vi "Add Stimulus Output Rows.vi"(8 "error in (no error)":errorcluster, 11 "Settings":T1 {"Processing Settings"."Test Parameters"."Allowed Tolerance (%) FS" format="%#_4g"; "Acq Settings"."Config Settings"."Simulated Sensor Injection" scale=0.0..100.0}) -> (0 "error out":errorcluster, 3 "Stimulus Outputs":T26)   [LabVIEW 2026, in "Settings.lvlib"]
uses:
  Settings.lvlib
  controls/UI/Stimulus Outputs Display.ctl
  controls/Controller/Stimulus Role.ctl
  controls/Controller/Stimulus Output Configuration.ctl
  controls/UI/Stimulus Output Display.ctl
  controls/UI/Measurement Role.ctl
  Acquisition/Instrument Specifications Cluster Configuration.ctl
  Acquisition/Acquisition.lvlib
  Acquisition/Instrument Specifications Configuration.ctl
  controls/UI/Config Settings.ctl
  controls/UI/Acq Settings.ctl
  controls/UI/Units Enum.ctl
  controls/UI/Signal Enum.ctl
  controls/Messaging Payloads/Sensor CoreData Cluster.ctl
  controls/Messaging Payloads/Sensor CoreData.ctl
  Processing/Test Parameters Cluster.ctl
  Processing/Test Parameters.ctl
  Processing/Processing_Engine.lvlib
  controls/UI/Direction.ctl
  controls/UI/Test Sequence Context.ctl
  Processing/Processing Settings.ctl
  controls/UI/Session Identfiers.ctl
  controls/UI/Test Sequence Enum.ctl
  controls/UI/Test Sequence State.ctl
  controls/UI/Test Sequence Settings.ctl
  controls/Controller/Controller Core Data.ctl
  controls/Controller/Stimulus Output.ctl
  controls/Controller/Stimulus Outputs.ctl
  controls/Controller/Stimulus Settings.ctl
  controls/UI/Settings Cluster.ctl
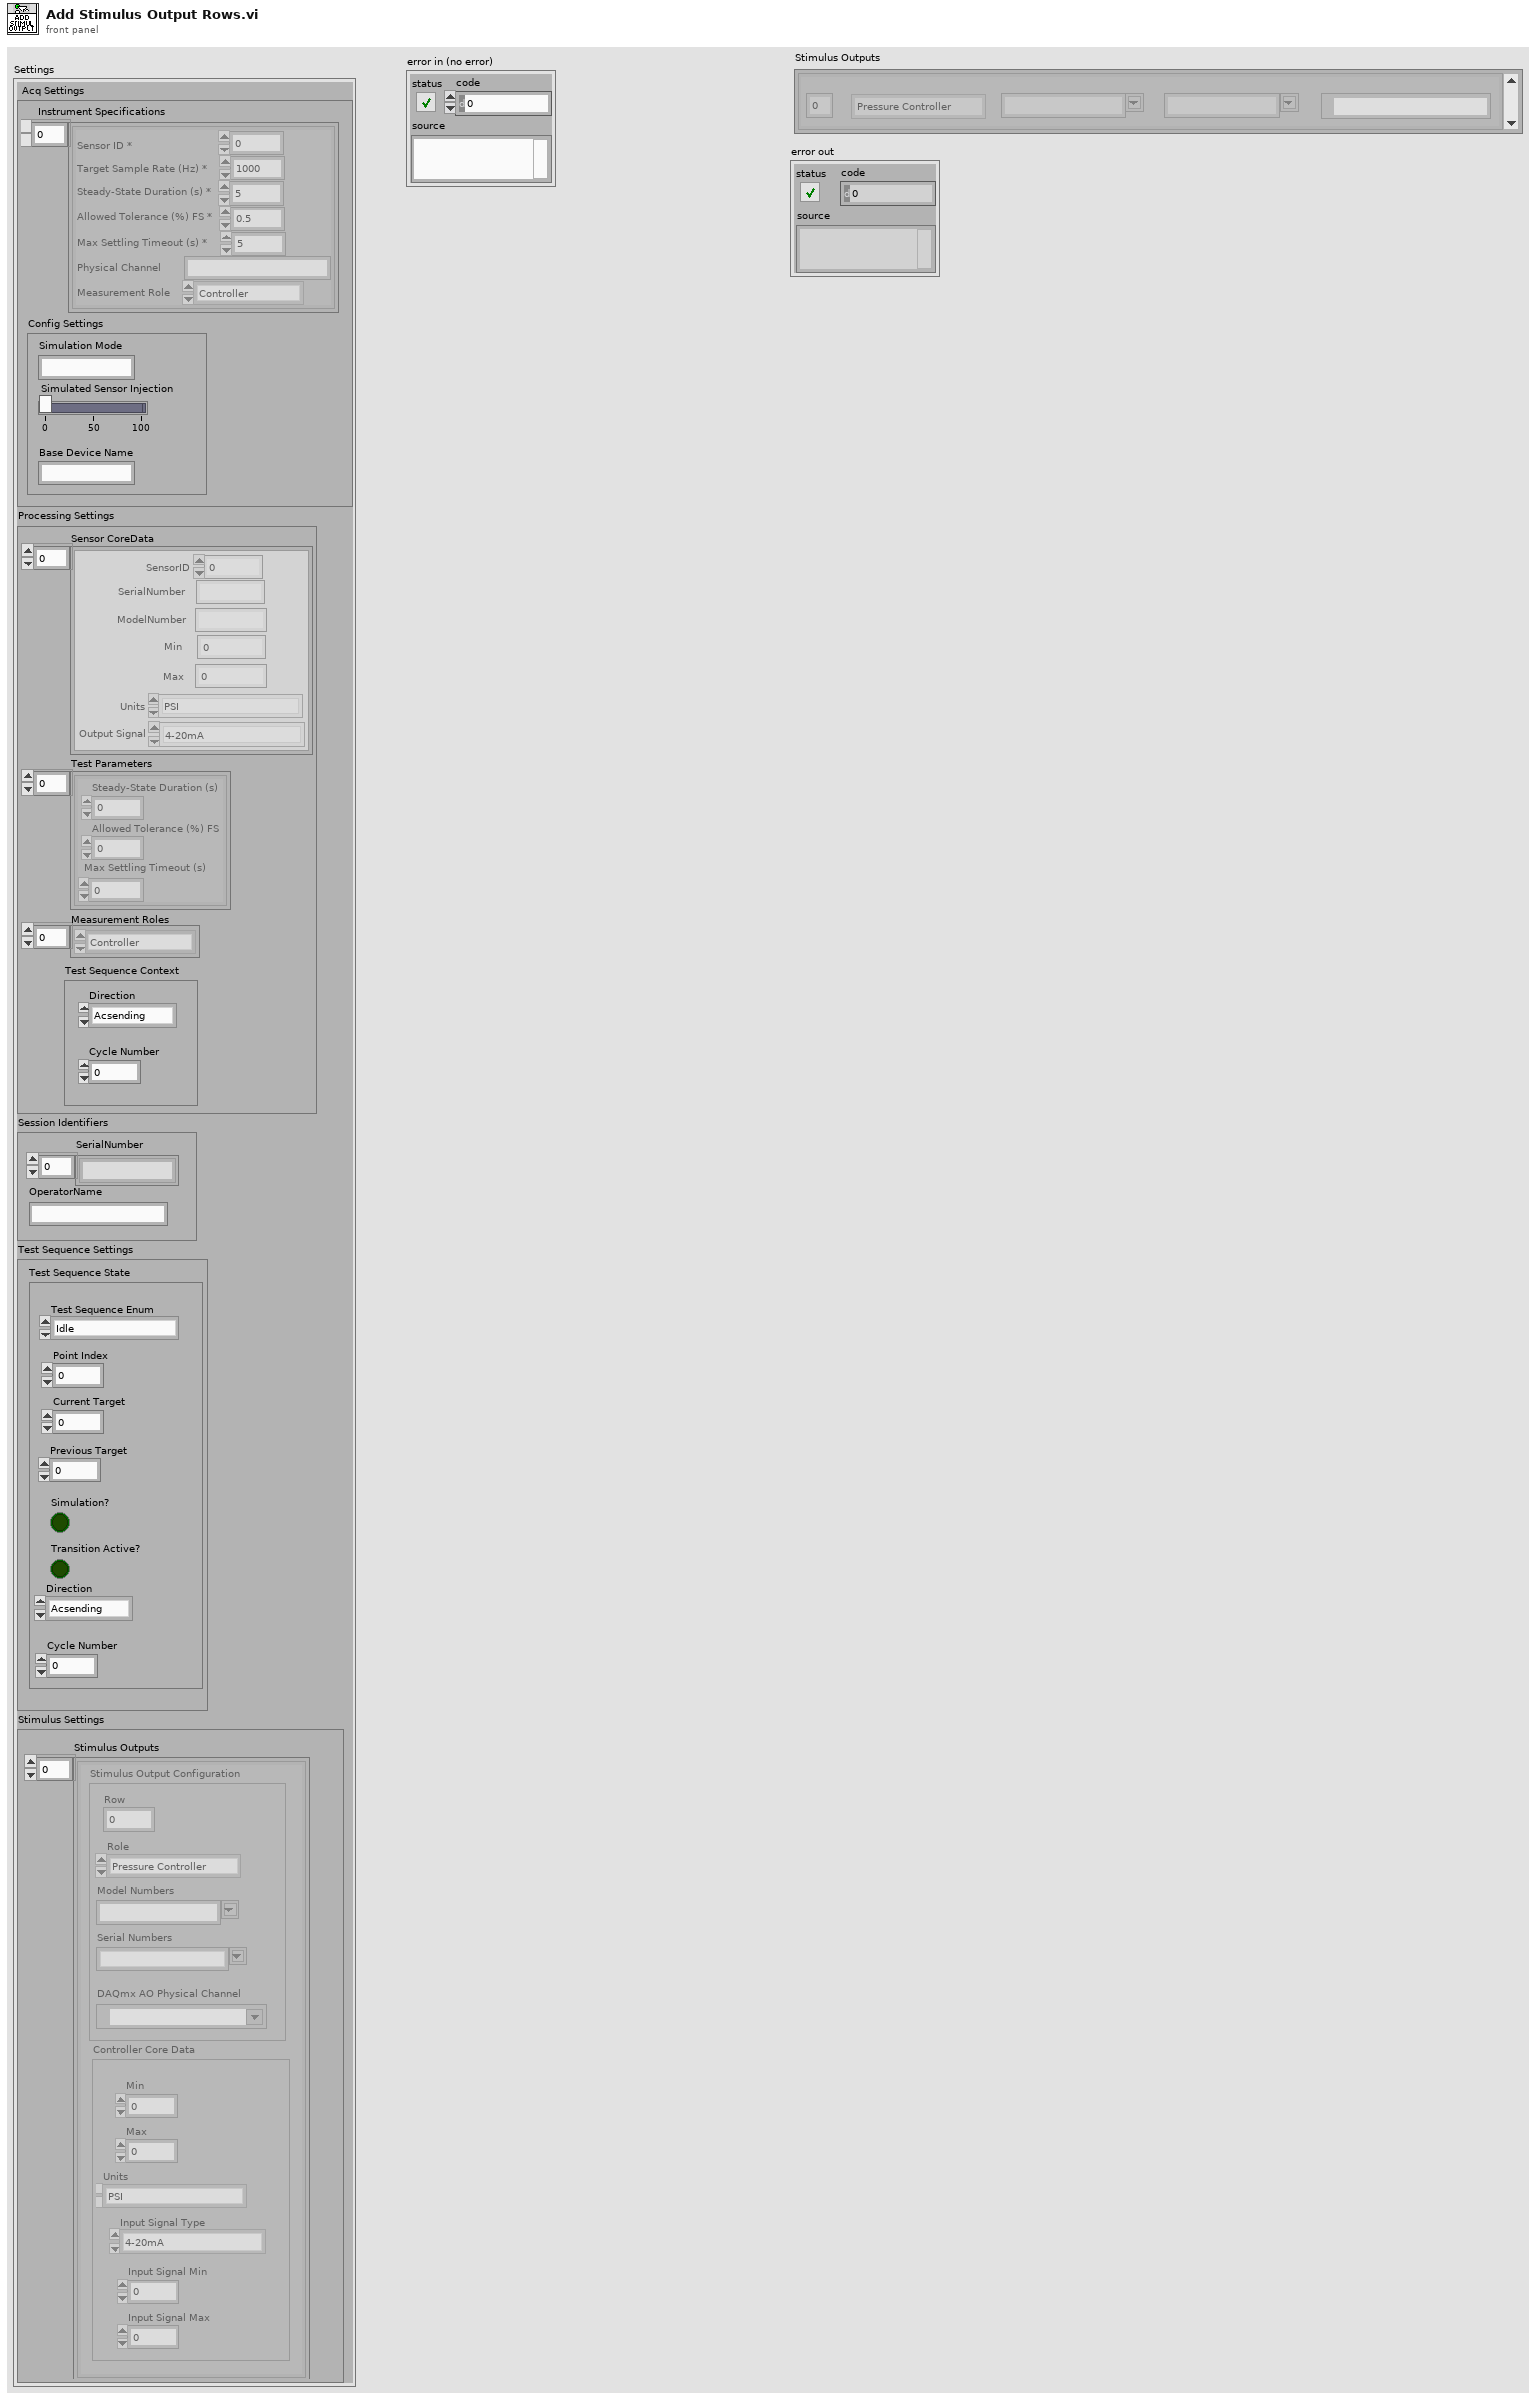
[diagram p1: front panel]
types:
  T1 = typedef "Settings Cluster.ctl" = cluster{"Acq Settings":T2, "Processing Settings":T7, "Session Identifiers":T16, "Test Sequence Settings":T17, "Stimulus Settings":T20}
  T2 = typedef "Acq Settings.ctl" = cluster{"Instrument Specifications":T3, "Config Settings":T6}
  T3 = typedef "Acquisition.lvlib/Instrument Specifications Configuration.ctl" = T4[]
  T4 = typedef "Acquisition.lvlib/Instrument Specifications Cluster Configuration.ctl" = cluster{"Sensor ID *":i32, "Target Sample Rate (Hz) *":dbl, "Steady-State Duration (s) *":i32, "Allowed Tolerance (%) FS *":dbl, "Max Settling Timeout (s) *":i32, "Physical Channel":string, "Measurement Role":T5}
  T5 = typedef "Settings.lvlib/Measurement Role.ctl" = enum16{"Controller", "Reference", "UUT", "Disable", "All"}
  T6 = typedef "Config Settings.ctl" = cluster{"Simulated Sensor Injection":dbl, "Base Device Name":string, "Simulation Mode":string}
  T7 = typedef "Processing_Engine.lvlib/Processing Settings.ctl" = cluster{"Sensor CoreData":T8, "Test Parameters":T12, "Measurement Roles":T5[], "Test Sequence Context":T14}
  T8 = typedef "Sensor CoreData.ctl" = T9[]
  T9 = typedef "Settings.lvlib/Sensor CoreData Cluster.ctl" = cluster{"SerialNumber":string, "ModelNumber":string, "Min":dbl, "Max":dbl, "Units":T10, "Output Signal":T11, "SensorID":i32}
  T10 = typedef "Units Enum.ctl" = enum16{"PSI", "Deg C", "kPa", "GPM"}
  T11 = typedef "Signal Enum.ctl" = enum16{"4-20mA", "0-10V", "Thermocouple Type K"}
  T12 = typedef "Processing_Engine.lvlib/Test Parameters.ctl" = T13[]
  T13 = typedef "Settings.lvlib/Test Parameters Cluster.ctl" = cluster{"Steady-State Duration (s)":i32, "Allowed Tolerance (%) FS":dbl, "Max Settling Timeout (s)":i32}
  T14 = typedef "Settings.lvlib/Test Sequence Context.ctl" = cluster{"Direction":T15, "Cycle Number":i32}
  T15 = typedef "Settings.lvlib/Direction.ctl" = enum16{"Acsending", "Descending"}
  T16 = typedef "Session Identfiers.ctl" = cluster{"SerialNumber":string[], "OperatorName":string}
  T17 = typedef "Test Sequence Settings.ctl" = cluster{"Test Sequence State":T18}
  T18 = typedef "Settings.lvlib/Test Sequence State.ctl" = cluster{"Test Sequence Enum":T19, "Point Index":i32, "Current Target":dbl, "Previous Target":dbl, "Simulation?":bool, "Direction":T15, "Transition Active?":bool, "Cycle Number":i32}
  T19 = typedef "Test Sequence Enum.ctl" = enum16{"Idle", "Start Point", "Point Complete", "Test Complete", "Abort Test", "Reset"}
  T20 = typedef "Settings.lvlib/Stimulus Settings.ctl" = cluster{"Stimulus Outputs":T21}
  T21 = typedef "Settings.lvlib/Stimulus Outputs.ctl" = T22[]
  T22 = typedef "Settings.lvlib/Stimulus Output.ctl" = cluster{"Controller Core Data":T23, "Stimulus Output Configuration":T24}
  T23 = typedef "Settings.lvlib/Controller Core Data.ctl" = cluster{"Min":dbl, "Max":dbl, "Units":T10, "Input Signal Type":T11, "Input Signal Min":dbl, "Input Signal Max":dbl}
  T24 = typedef "Settings.lvlib/Stimulus Output Configuration.ctl" = cluster{"DAQmx AO Physical Channel":tag, "Role":T25, "Model Numbers":string, "Serial Numbers":string, "Row":i32}
  T25 = typedef "Stimulus Role.ctl" = enum16{"Pressure Controller", "Temperature Controller"}
  T26 = typedef "Settings.lvlib/Stimulus Outputs Display.ctl" = T27[]
  T27 = typedef "Settings.lvlib/Stimulus Output Display.ctl" = cluster{"DAQmx AO Physical Channel":tag, "Role":T25, "Model Numbers":string, "Serial Numbers":string, "Row":i32}
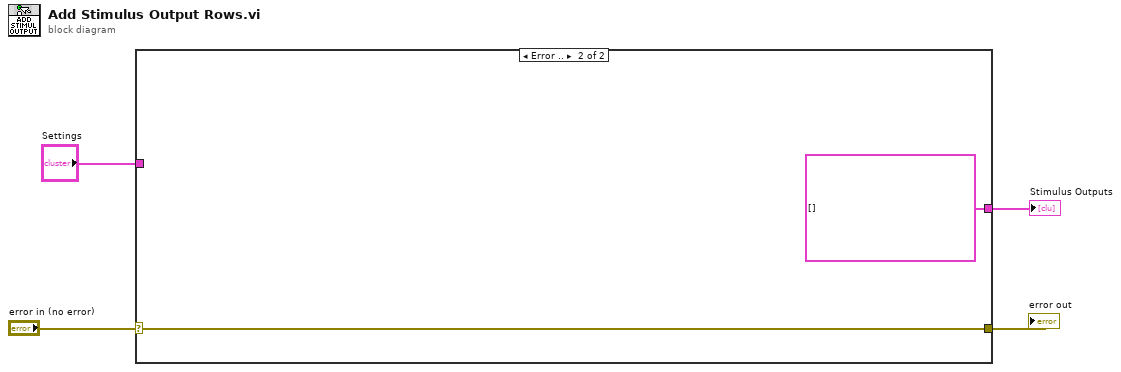
[diagram p0: block diagram]
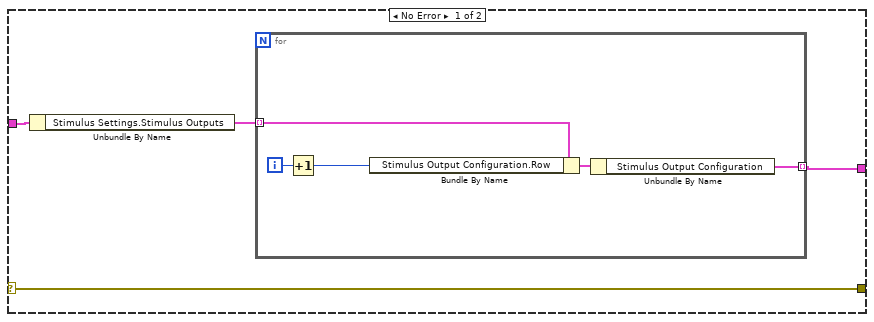
[diagram p2: hidden frame]
diagram:
  n1 = case shown="Error .." "error in (no error)" {
    selector: "error in (no error)" -> [w8 w15]
    tunnel: [w8 w15] -> w3
    tunnel: "Settings" -> [w7 _]
    tunnel: [w5 T24[] []] -> w1
    frame No Error {
      n2 = Unbundle By Name(w7) -> ("Stimulus Settings.Stimulus Outputs"=w6:T21)
      n3 = for {
        tunnel: w6 -> [w11] mode=indexing
        tunnel: [w9] -> w5 mode=indexing
        i -> [w13]
        n4 = Increment(x=w13) -> (x+1=w12:i32)
        n5 = Bundle By Name(cluster=w11, "Stimulus Output Configuration.Row"=w12) -> (w10:T22)
        n6 = Unbundle By Name(w10) -> ("Stimulus Output Configuration"=w9:T24)
      }
    }
    frame Error {
    }
  }
  "error out" <- w3
  "Stimulus Outputs" <- w1
